vi "Voltmeter.vi"(1 "Action":T4=enum."Identify", 2 "Parameters":variant) -> (6 "Output":variant, 7 "Stop":bool)   [LabVIEW 2024]
doc: "This VI reads a single reading from a Keithley 2001 multimeter. The stop boolean is always false. If no reading is obtained a single zero is returned.\nScott Hannahs, NHMFL-FSU, Nov 1993"
uses:
  Sub Controls/Instrument Actions.ctl
  Sub Controls/Instrument Match.ctl
  Sub Controls/Public.ctl
  Sub Controls/Factory Reset.ctl
  Sub Controls/Scan Input.ctl
  Sub Controls/Scan Output.ctl
  Sub Controls/Instrument IDN.ctl
  Sub Controls/User Event Command.ctl
panel:
  in  "Factory Reset":T1
  in  "Elements":bool
  in  "Mode Sourcemeter":enum32{"Voltage", "Current", "Both"}(radio)
  out "Title":string
  in  "Public":T2
  in  "Address":u16(ring)
  out "Model":string
  in  "Instruments":T3[](array[typedef])=[{"Model"="34401", "Manufacturer"="HEWLETT-PACKARD", "Term Character"="", "Wait Time (mS)"=0, "Wait for SRQ"=FALSE, "Type"="Voltmeter"}, {"Model"="MODEL 182", "Manufacturer"="KEITHLEY INSTRUMENTS", "Term Character"="", "Wait Time (mS)"=0, "Wait for SRQ"=FALSE, "Type"="Voltmeter"}, {"Model"="MODEL 200[012]", "Manufacturer"="KEITHLEY INSTRUMENTS", "Term Character"="", "Wait Time (mS)"=0, "Wait for SRQ"=FALSE, "Type"="Voltmeter"}, {"Model"="MODEL 6221[A]*", "Manufacturer"="KEITHLEY INSTRUMENTS", "Term Character"="", "Wait Time (mS)"=0, "Wait for SRQ"=FALSE, "Type"="Voltmeter"}, {"Model"="MODEL 2420", "Manufacturer"="KEITHLEY INSTRUMENTS", "Term Character"="", "Wait Time (mS)"=0, "Wait for SRQ"=FALSE, "Type"="Voltmeter"}, {"Model"="MODEL 2182[A]*", "Manufacturer"="KEITHLEY INSTRUMENTS", "Term Character"="", "Wait Time (mS)"=0, "Wait for SRQ"=FALSE, "Type"="Voltmeter"}, {"Model"="MODEL 6517[AB]", "Manufacturer"="KEITHLEY INSTRUMENTS", "Term Character"="", "Wait Time (mS)"=0, "Wait for SRQ"=FALSE, "Type"="Electrometer"}, {"Model"="MODEL 6430", "Manufacturer"="KEITHLEY INSTRUMENTS", "Term Character"="", "Wait Time (mS)"=0, "Wait for SRQ"=FALSE, "Type"="Sourcemeter"}, {"Model"="5313[12]A", "Manufacturer"="HEWLETT-PACKARD", "Term Character"="", "Wait Time (mS)"=0, "Wait for SRQ"=FALSE, "Type"="Counter"}, {"Model"="MODEL 2450", "Manufacturer"="KEITHLEY INSTRUMENTS", "Term Character"="", "Wait Time (mS)"=0, "Wait for SRQ"=FALSE, "Type"="Sourcemeter"}, {"Model"="MODEL DMM7510", "Manufacturer"="KEITHLEY INSTRUMENTS", "Term Character"="", "Wait Time (mS)"=0, "Wait for SRQ"=FALSE, "Type"="Voltmeter"}]
  out "Measurement":dbl[](array[numeric]) format="%^_7e"
  in  "VISA resource name":refnum<visa-resource-name>
  # "Term Char"
  # "Wait Time (mS)"
  # "Wait for SRQ?"
  # "Type"
  # "Manufacturer"
  # "Model"
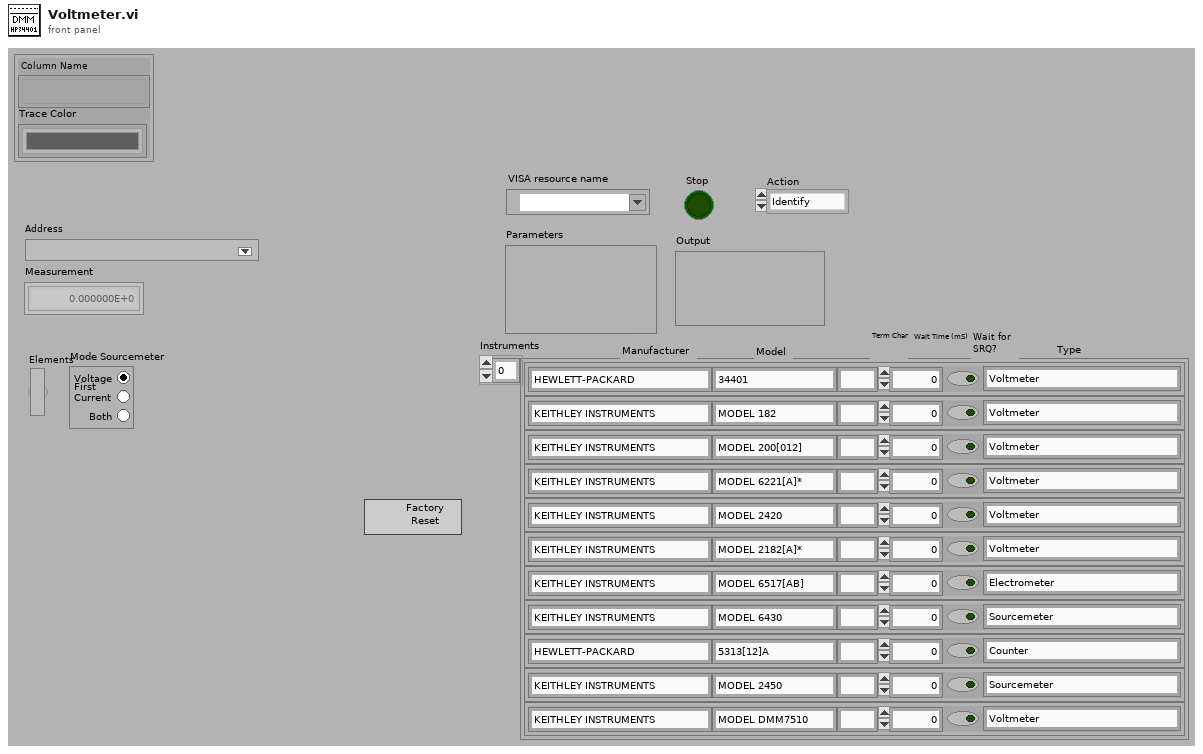
[diagram p1: front panel]
types:
  T1 = typedef "Factory Reset.ctl" = bool
  T2 = typedef "Public.ctl" = cluster{"Column Name":string[], "Trace Color":u32[]}
  T3 = typedef "Instrument Match.ctl" = cluster{"Model":string, "Manufacturer":string, "Term Character":string, "Wait Time (mS)":u32, "Wait for SRQ":bool, "Type":string}
  T4 = typedef "Instrument Actions.ctl" = enum16{"Scan", "Identify", "New", "Configure", "Initialize", "Test", "Read", "Close"}
  T5 = typedef "Scan Output.ctl" = cluster{"Manufacturer":string, "Model":string, "Info":string, "Revision":string, "error out":errorcluster}
  T6 = typedef "Scan Input.ctl" = cluster{"VISA resource name":refnum<visa-resource-name>, "ID String in":string}
  T7 = typedef "Instrument IDN.ctl" = cluster{"VISA Address":string, "Status":u16, "Manufacturer":string, "Model":string, "Info":string, "Info 2":string, "Misc Data":variant}
  T8 = typedef "User Event Command.ctl" = enum32{"Stop Config"}
  T9 = typedef "Instrument Properties.ctl" = cluster{"Public":T2, "Private":T10}
  T10 = typedef "Private.ctl" = cluster{"Path":path, "VI Refnum":T11, "Name":string, "# of Values":i32, "Scale Factors":dbl[], "Display":T12[], "Offset":dbl[]}
  T11 = typedef "Instrument Ref.ctl" = refnum<vi>
  T12 = typedef "SystemCheckBox-resize.ctl" = bool
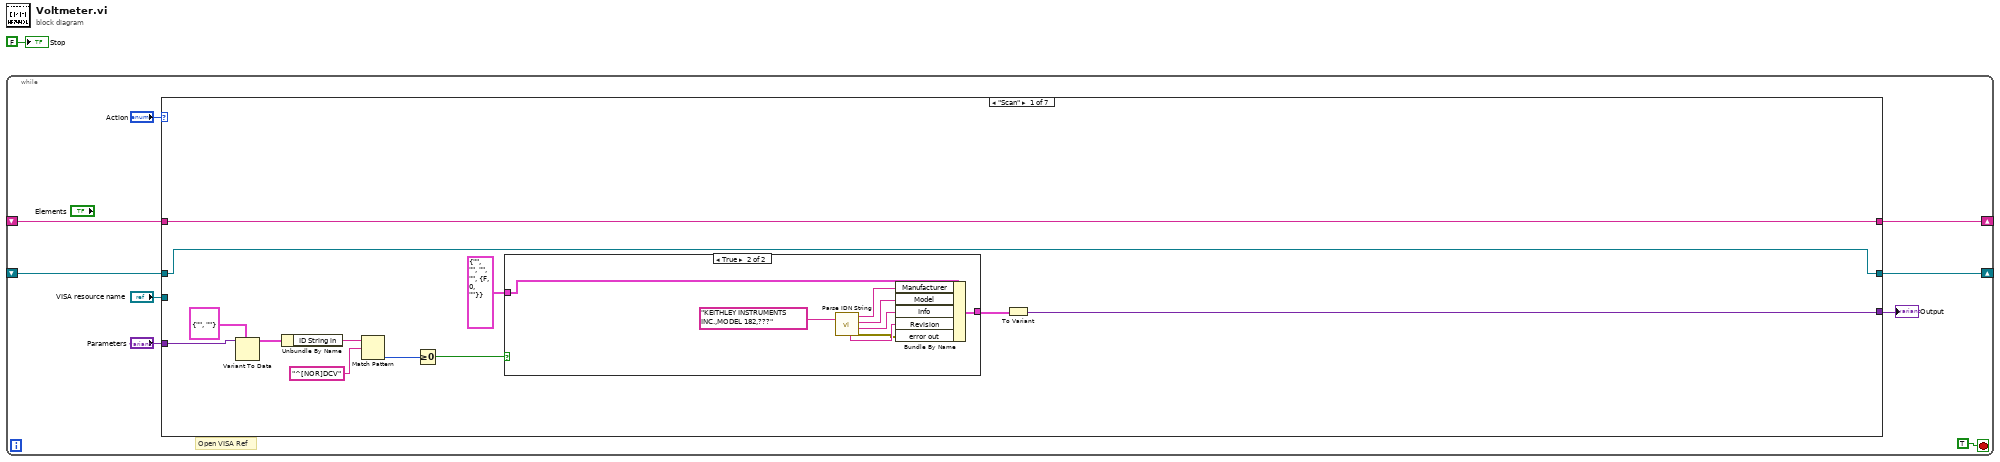
[diagram p0: block diagram]
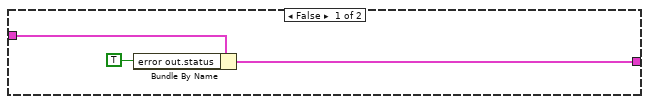
[diagram p2: hidden frame]
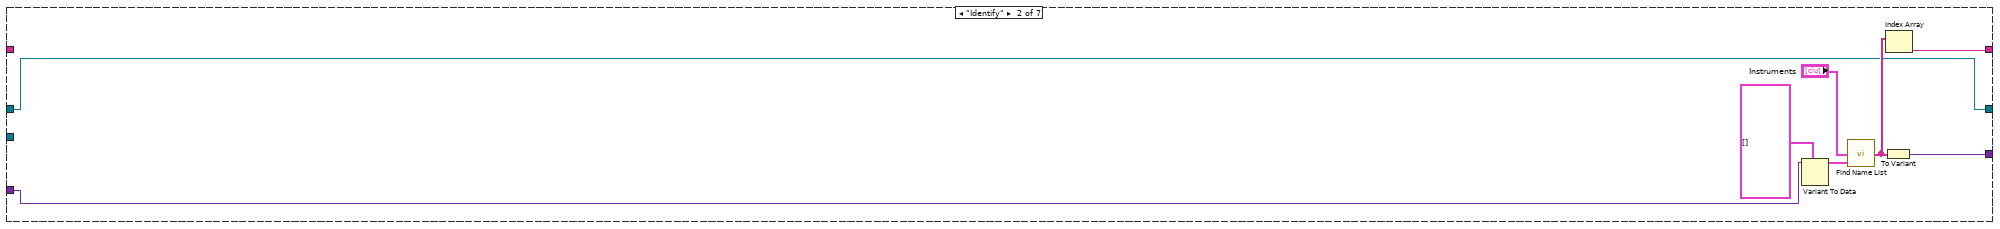
[diagram p3: hidden frame]
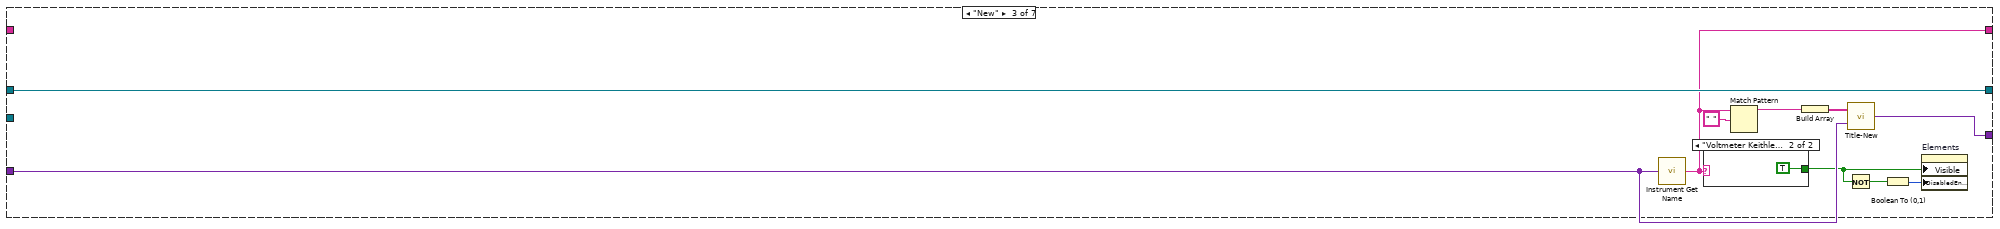
[diagram p4: hidden frame]
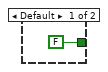
[diagram p5: hidden frame]
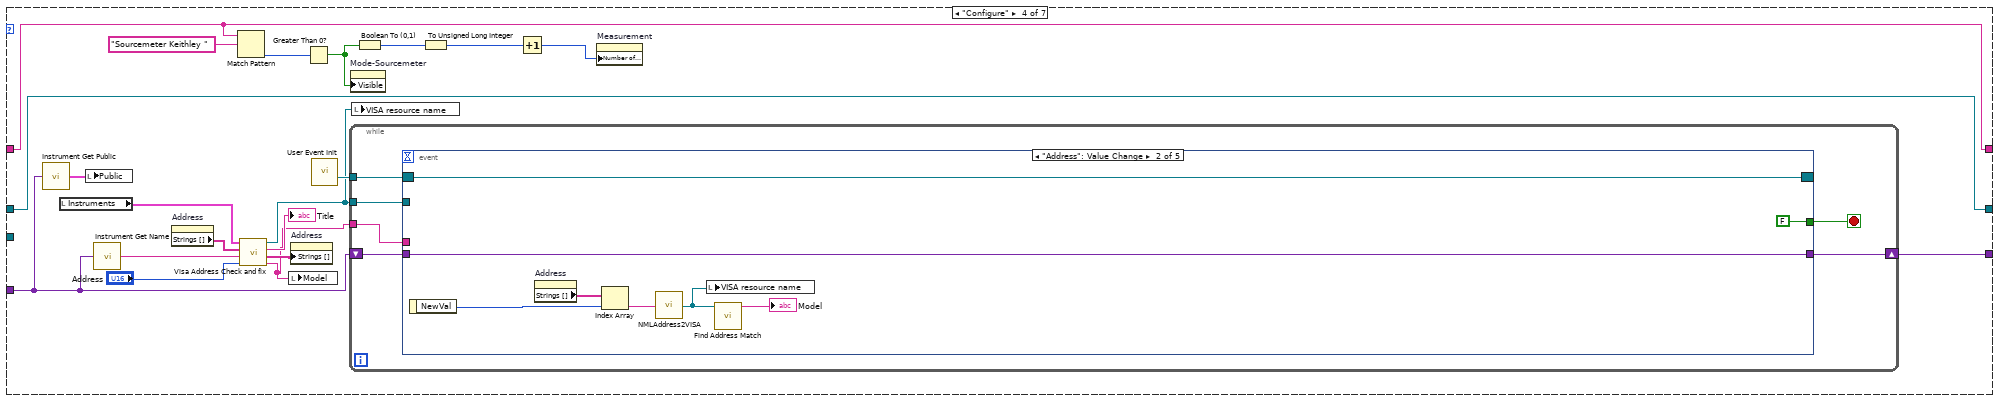
[diagram p6: hidden frame]
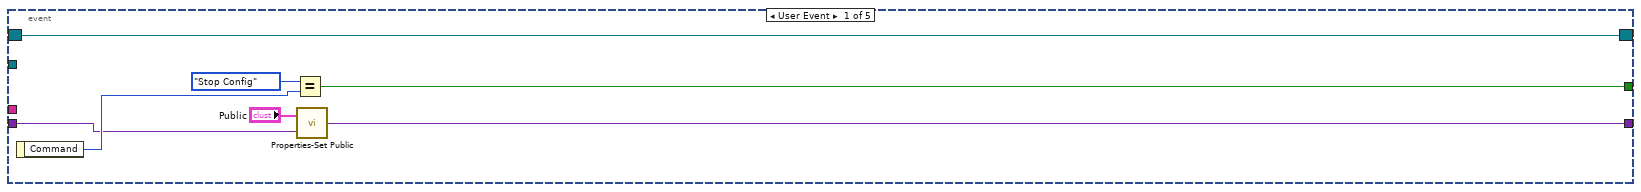
[diagram p7: hidden frame]
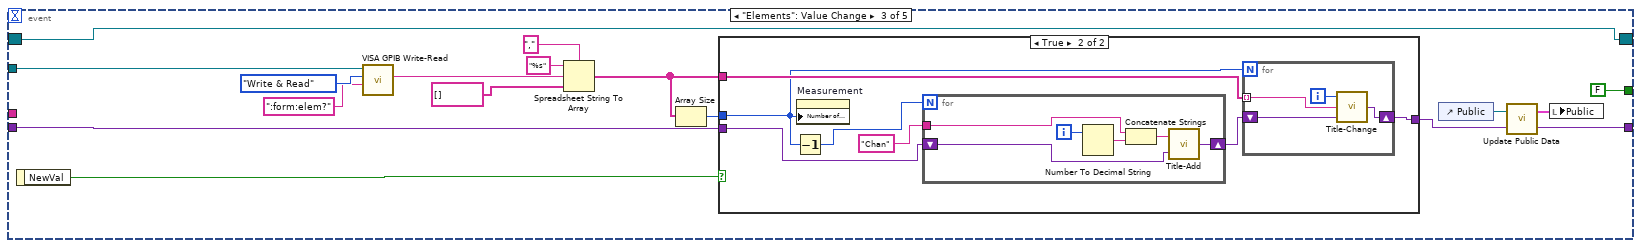
[diagram p8: hidden frame]
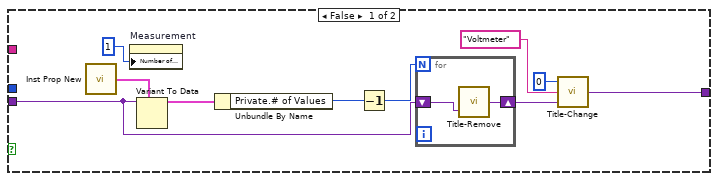
[diagram p9: hidden frame]
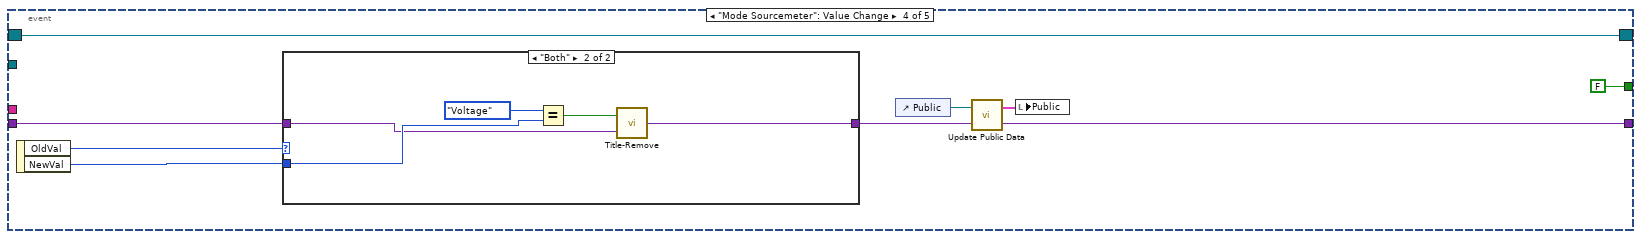
[diagram p10: hidden frame]
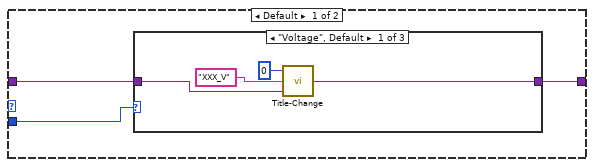
[diagram p11: hidden frame]
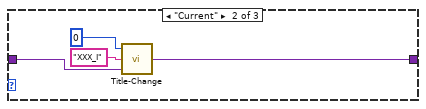
[diagram p12: hidden frame]
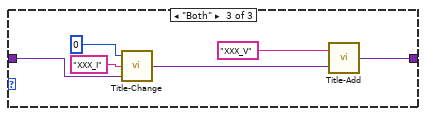
[diagram p13: hidden frame]
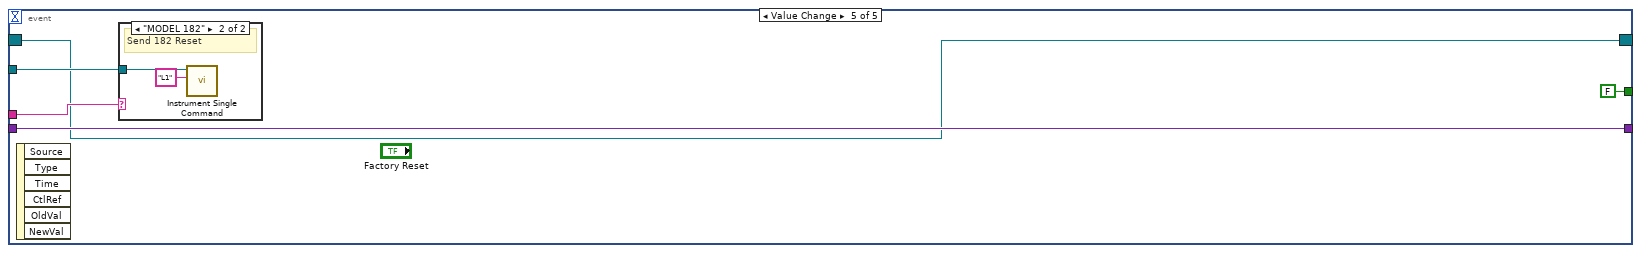
[diagram p14: hidden frame]
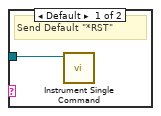
[diagram p15: hidden frame]
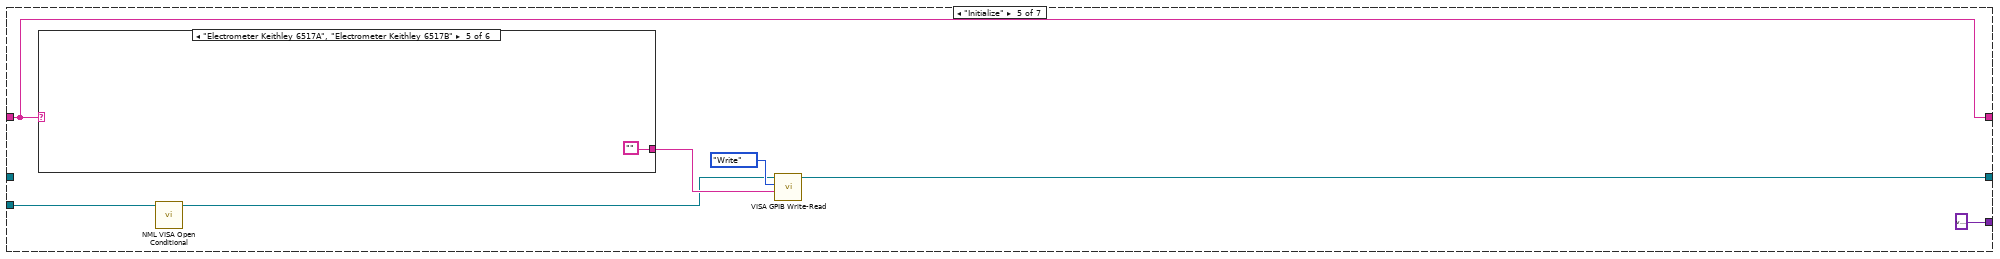
[diagram p16: hidden frame]
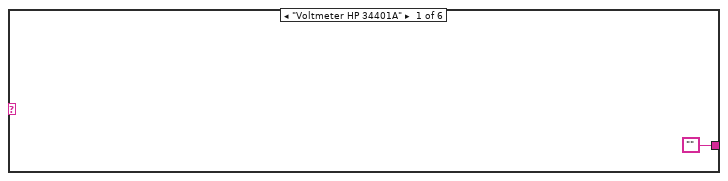
[diagram p17: hidden frame]
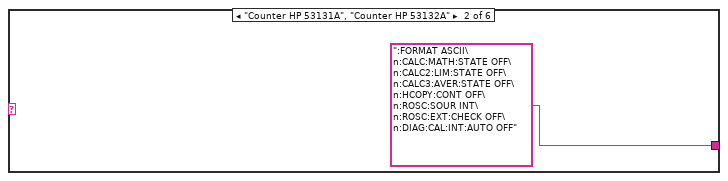
[diagram p18: hidden frame]
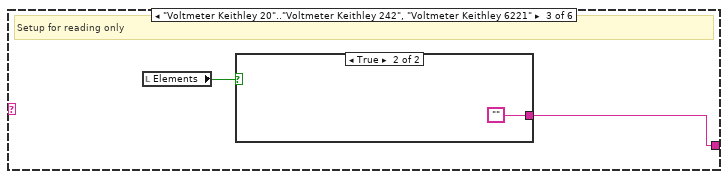
[diagram p19: hidden frame]
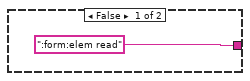
[diagram p20: hidden frame]
diagram:
  n1 = while {
    shift-right: [w6] -> _
    shift-left: _ -> [w5]
    shift-right: [w3] -> _
    shift-left: _ -> [w2]
    stop <- TRUE stop-if-true
    # "Open VISA Ref"
    n2 = case shown="\"Scan\"" "Action" {
      tunnel: [w15 w41 w51 w68 variant ("Variant") w203 variant ("Variant")] -> w8
      tunnel: "VISA resource name" -> [_ _ _ _ w186 _ _]
      tunnel: [w14 w36 w45 w59 w183 w197 w240] -> w6
      tunnel: w5 -> [w14 _ _ w59 w183 w197 w240]
      tunnel: "Parameters" -> [w22 w40 w49 w65 _ _ _]
      tunnel: [w11 w34 w50 w66 w182 w201 refnum<visa-resource-name> refnum ("Open VISA Resource name")] -> w3
      tunnel: w2 -> [w11 w34 w50 w66 _ w202 w238]
      frame "Scan" {
        n3 = Variant To Data(type=T6 {"VISA resource name"="", "ID String in"=""} ("Scan Input"), Variant=w22) -> (data=w20:T6)  [unwired: 1 in, 1 out]
        n4 = Unbundle By Name(w20) -> ("ID String in"=w17:string)
        n5 = Match Pattern(string=w17, regular expression="^[NOR]DCV") -> (offset past match=w19:i32)  [unwired: 1 in, 3 out]
        n6 = Greater Or Equal To 0?(x=w19) -> (x >= 0?=w16:bool)
        n7 = case shown="True" w16 {
          tunnel: T5 {"Manufacturer"="", "Model"="", "Info"="", "Revision"="", "error out"={"status"=FALSE, "code"=0, "source"=""}} ("Scan Output") -> [w24 w33]
          tunnel: [w25 w32] -> w12
          frame False {
            n8 = Bundle By Name(cluster=w24, "error out.status"=TRUE) -> (w25:T5)
          }
          frame True {
            n9 = call "Parse IDN String.vi"("IDN String"="KEITHLEY INSTRUMENTS INC.,MODEL 182,???") -> ("error out"=w29:errorcluster, "Info"=w28:string, "Model"=w27:string, "Manufacturer"=w26:string, "Revision"=w30:string)  [unwired: 1 in]
            n10 = Bundle By Name(cluster=w33, "Manufacturer"=w26, "Model"=w27, "Info"=w28, "Revision"=w30, "error out"=w29) -> (w32:T5)
          }
        }
        n11 = To Variant(anything=w12) -> (Variant=w15:variant)
      }
      frame "Identify" {
        n12 = Variant To Data(type=T7[] [], Variant=w40) -> (data=w38:T7[])  [unwired: 1 in, 1 out]
        n13 = call "Find Name List.vi"("Bus Scan"=w38, "Instruments"="Instruments") -> ("Names"=w35:string[])  [unwired: 1 in]
        n14 = Index Array(array=w35) -> (element=w36:string)  [unwired: 1 in]
        n15 = To Variant(anything=w35) -> (Variant=w41:variant)
      }
      frame "New" {
        n16 = call "Instrument Get Name.vi"("Parameters"=w49) -> ("Type"=w45:string)
        n17 = case shown="\"Voltmeter Keithley 6221\"" w45 {
          tunnel: [FALSE ("Visible") TRUE ("Visible")] -> w44
          frame Default {
          }
          frame "Voltmeter Keithley 6221" {
          }
        }
        n18 = Match Pattern(string=w45, regular expression=" ") -> (before substring=w47:string)  [unwired: 1 in, 3 out]
        n19 = Build Array(w47) -> (w48:string[])
        n20 = Not(x=w44) -> (.not. x?=w42:bool)
        n21 = call "Title-New.vi"("Parameters"=w49, "Array"=w48) -> ("Instrument Prop"=w51:variant)
        n22 = Boolean To (0,1)(Boolean=w42) -> (0, 1=w43:i16)
        n23 = property on="Elements" class="Bool (strict)"("Visible"=w44, "DisabledEnum"=w43) -> ()  [unwired: 2 in, 2 out]
      }
      frame "Configure" {
        n24 = call "Instrument Get Public.vi"("Variant"=w65) -> ("Public"=w69:T2)
        n25 = local read "Instruments"() -> (w70:T3[])
        n26 = local write "Public"(w69) -> ()
        n27 = call "Instrument Get Name.vi"("Parameters"=w65) -> ("Type"=w64:string)
        n28 = property on="Address" class="Ring (strict)"() -> ("Strings []"=w71:string[])  [unwired: 2 in, 2 out]
        n29 = Match Pattern(string=w59, regular expression="Sourcemeter Keithley " ("y")) -> (offset past match=w57:i32)  [unwired: 1 in, 3 out]
        n30 = call "Visa Address Check and fix.vi"("Address"="Address", "Name"=w64, "NML Addresses"=w71, "Instruments"=w70) -> ("Model"=w54:string, "NML Addresses"=w73:string[], "Title"=→"Title":string, "VISA resource name"=w55:refnum<visa-resource-name>)  [unwired: 2 out]
        n31 = local write "Model"(w54) -> ()
        n32 = property on="Address" class="Ring (strict)"("Strings []"=w73) -> ()  [unwired: 2 in, 2 out]
        n33 = Greater Than 0?(x=w57) -> (x > 0?=w56:bool)
        n34 = call "User Event Init.vi"() -> ("Event Registration Refnum"=w67:refnum<event-registration>)  [unwired: 14 in, 1 out]
        n35 = while {
          tunnel: w67 -> [w76]
          shift-right: [w79] -> w68
          shift-left: w65 -> [w77]
          tunnel: w55 -> [w75]
          tunnel: w54 -> [w74]
          stop <- w78 stop-if-true
          n36 = event shown="[1] \"Address\": Value Change" {
            selector: w76 -> [w80 w88 w108 w149 w172]
            dyn-events: [w80 w88 w108 w149 w172] -> _
            timeout: _ -> [_ _ _ _ _]
            tunnel: [w84 w89 w105 w143 w174] -> w79
            tunnel: [w82 FALSE FALSE FALSE FALSE] -> w78
            tunnel: w77 -> [w85 w89 w111 w145 w174]
            tunnel: w75 -> [_ _ w101 _ w176]
            tunnel: w74 -> [_ _ _ _ w175]
            event User Event {
              n37 = event-data() -> ("Command"=w86:T8)  [unwired: 1 in]
              n38 = Equal?(x=User_Event_Command."Stop Config", y=w86) -> (x = y?=w82:bool)
              n39 = call "Properties-Set Public.vi"("Variant"=w85, "New Public"="Public") -> ("Variant 2"=w84:variant)
            }
            event "Address": Value Change {
              n40 = event-data() -> ("NewVal"=w94:u16)  [unwired: 1 in]
              n41 = property on="Address" class="Ring (strict)"() -> ("Strings []"=w91:string[])  [unwired: 2 in, 2 out]
              n42 = Index Array(array=w91, index=w94) -> (element=w92:string)
              n43 = call "NMLAddress2VISA.vi"("NML Address"=w92) -> ("VISA resource name"=w87:refnum<visa-resource-name>)
              n44 = local write "VISA resource name"(w87) -> ()
              n45 = call "Find Address Match.vi"("VISA resource name"=w87) -> ("Model"=→"Model":string)  [unwired: 3 in, 3 out]
            }
            event "Elements": Value Change {
              n46 = event-data() -> ("NewVal"=w110:bool)  [unwired: 1 in]
              n47 = call "VISA GPIB Write-Read.vi"("Command"=":form:elem?", "Action"=enum16{"Write", "Read", "Write & Read"}."Write & Read", "VISA resource name"=w101) -> ("String Returned"=w100:string)  [unwired: 5 in, 3 out]
              n48 = Spreadsheet String To Array(delimiter (Tab)=",", format string="%s", spreadsheet string=w100, array type (2D Dbl)=string[] [] ("array")) -> (array=w95:string[])
              n49 = Array Size(array=w95) -> (size(s)=w97:i32)
              n50 = case shown="True" w110 {
                tunnel: w111 -> [w118 w129]
                tunnel: [w115 w125] -> w106
                tunnel: w97 -> [_ w126]
                tunnel: w95 -> [_ w127]
                frame False {
                  n51 = call "Inst Prop New.vi"() -> ("Instrument Prop Out"=w121:T9)
                  n52 = property on="Measurement" class="Arr (strict)"("Number of Columns"=u32 1) -> ()  [unwired: 2 in, 2 out]
                  n53 = Variant To Data(type=w121, Variant=w118) -> (data=w120:T9)  [unwired: 1 in, 1 out]
                  n54 = Unbundle By Name(w120) -> ("Private.# of Values"=w119:i32)
                  n55 = Decrement(x=w119) -> (x-1=w113:i32)
                  n56 = for {
                    N: w113 -> [_]
                    shift-right: [w123] -> w116
                    shift-left: w118 -> [w122]
                    n57 = call "Title-Remove.vi"("Parameters"=w122) -> ("Variant"=w123:variant)  [unwired: 1 in]
                  }
                  n58 = call "Title-Change.vi"("Parameters"=w116, "New Title"="Voltmeter", "Index"=0) -> ("Variant"=w115:variant)
                }
                frame True {
                  n59 = Decrement(x=w126) -> (x-1=w130:i32)
                  n60 = property on="Measurement" class="Arr (strict)"("Number of Columns"=w126) -> ()  [unwired: 2 in, 2 out]
                  n61 = for {
                    N: w130 -> [_]
                    tunnel: "Chan" ("String") -> [w139]
                    shift-right: [w140] -> w124
                    shift-left: w129 -> [w135]
                    i -> [w137]
                    n62 = Number To Decimal String(number=w137) -> (decimal integer string=w136:string)  [unwired: 1 in]
                    n63 = Concatenate Strings(w139, w136) -> (w138:string)
                    n64 = call "Title-Add.vi"("Parameters"=w135, "String"=w138) -> ("Variant"=w140:variant)
                  }
                  n65 = for {
                    N: w126 -> [_]
                    tunnel: w127 -> [w133] mode=indexing
                    shift-right: [w132] -> w125
                    shift-left: w124 -> [w131]
                    i -> [w134]
                    n66 = call "Title-Change.vi"("Parameters"=w131, "New Title"=w133, "Index"=w134) -> ("Variant"=w132:variant)
                  }
                }
              }
              n67 = control-ref of="Public"() -> (w104:refnum<vi>)
              n68 = call "Update Public Data.vi"("Variant In"=w106, "Public 2"=w104) -> ("Variant Out"=w105:variant, "Public"=w107:T2)
              n69 = local write "Public"(w107) -> ()
            }
            event "Mode Sourcemeter": Value Change {
              n70 = event-data() -> ("OldVal"=w147:enum32{"Voltage", "Current", "Both"}, "NewVal"=w146:enum32{"Voltage", "Current", "Both"})  [unwired: 1 in]
              n71 = case shown="\"Both\"" w147 {
                tunnel: w146 -> [w152 w170]
                tunnel: w145 -> [w151 w167]
                tunnel: [w150 w171] -> w144
                frame Default {
                  n72 = case shown="\"Voltage\", Default" w152 {
                    tunnel: w151 -> [w156 w157 w164]
                    tunnel: [w153 w158 w162] -> w150
                    frame "Voltage", Default {
                      n73 = call "Title-Change.vi"("Parameters"=w156, "New Title"="XXX_V", "Index"=0) -> ("Variant"=w153:variant)
                    }
                    frame "Current" {
                      n74 = call "Title-Change.vi"("Parameters"=w157, "New Title"="XXX_I", "Index"=0) -> ("Variant"=w158:variant)
                    }
                    frame "Both" {
                      n75 = call "Title-Change.vi"("Parameters"=w164, "New Title"="XXX_I", "Index"=0) -> ("Variant"=w163:variant)
                      n76 = call "Title-Add.vi"("Parameters"=w163, "String"="XXX_V") -> ("Variant"=w162:variant)
                    }
                  }
                }
                frame "Both" {
                  n77 = Equal?(x=enum32{"Voltage", "Current", "Both"}."Voltage", y=w170) -> (x = y?=w168:bool)
                  n78 = call "Title-Remove.vi"("Parameters"=w167, "Remove First"=w168) -> ("Variant"=w171:variant)
                }
              }
              n79 = control-ref of="Public"() -> (w141:refnum<vi>)
              n80 = call "Update Public Data.vi"("Variant In"=w144, "Public 2"=w141) -> ("Variant Out"=w143:variant, "Public"=w142:T2)
              n81 = local write "Public"(w142) -> ()
            }
            event Value Change {
              n82 = event-data() -> ()  [unwired: 1 in, 6 out]
              n83 = case shown="\"MODEL 182\"" w175 {
                tunnel: w176 -> [w177 w179]
                frame Default {
                  # "Send Default \"*RST\""
                  n84 = call "Instrument Single Command.vi"("VISA Name"=w177) -> ()  [unwired: 10 in, 1 out]
                }
                frame "MODEL 182" {
                  # "Send 182 Reset"
                  n85 = call "Instrument Single Command.vi"("Reset Command"="L1", "VISA Name"=w179) -> ()  [unwired: 9 in, 1 out]
                }
              }
            }
          }
        }
        n86 = property on="Mode-Sourcemeter" class="RadioBtnsControl (strict)"("Visible"=w56) -> ()  [unwired: 2 in, 2 out]
        n87 = local write "VISA resource name"(w55) -> ()
        n88 = Boolean To (0,1)(Boolean=w56) -> (0, 1=w62:i16)
        n89 = To Unsigned Long Integer(number=w62) -> (unsigned 32bit integer=w60:u32)
        n90 = Increment(x=w60) -> (x+1=w61:u32)
        n91 = property on="Measurement" class="Arr (strict)"("Number of Columns"=w61) -> ()  [unwired: 2 in, 2 out]
      }
      frame "Initialize" {
        n92 = case shown="\"Electrometer Keithley 6517A\", \"Electrometer Keithley 6517B\"" w183 {
          tunnel: ["" ":FORMAT ASCII\n:CALC:MATH:STATE OFF\n:CALC2:LIM:STATE OFF\n:CALC3:AVER:STATE OFF\n:HCOPY:CONT OFF\n:ROSC:SOUR INT\n:ROSC:EXT:CHECK OFF\n:DIAG:CAL:INT:AUTO OFF" w190 ":form:elem VOLT,CURR" "" ""] -> w184
          frame "Voltmeter HP 34401A" {
          }
          frame "Counter HP 53131A", "Counter HP 53132A" {
          }
          frame "Voltmeter Keithley 20".."Voltmeter Keithley 242", "Voltmeter Keithley 6221" {
            # "Setup for reading only"
            n93 = local read "Elements"() -> (w189:bool)
            n94 = case shown="True" w189 {
              tunnel: [":form:elem read" ""] -> w190
              frame False {
              }
              frame True {
              }
            }
          }
          frame "Sourcemeter Keithley 6430" {
          }
          frame "Electrometer Keithley 6517A", "Electrometer Keithley 6517B" {
          }
          frame "Voltmeter Keithley 182", Default {
          }
        }
        n95 = call "NML VISA Open Conditional.vi"("VISA resource name"=w186) -> ("dup VISA Session"=w180:refnum<visa-resource-name>)  [unwired: 8 in, 2 out]
        n96 = call "VISA GPIB Write-Read.vi"("Command"=w184, "Action"=enum16{"Write", "Read", "Write & Read"}."Write", "VISA resource name"=w180) -> ("dup VISA Session"=w182:refnum<visa-resource-name>)  [unwired: 5 in, 3 out]
      }
      frame "Test", "Read" {
        n97 = case shown="\"Sourcemeter Keithley 2450\"" w197 {
          tunnel: ["read?" "fetc?" "Sens:data:latest?" w219 w229 ""] -> w200
          tunnel: [u32 0 ("wait (mS)") u32 50 ("wait (mS)") u32 0 ("wait (mS)") u32 0 ("wait (mS)") u32 0 ("wait (mS)") u32 0 ("wait (mS)")] -> w196
          frame "Voltmeter HP 34401A", "Voltmeter Keithley DMM7510" {
          }
          frame "Counter HP 53131A", "Counter HP 53132A" {
          }
          frame "Electrometer Keithley 6517A", "Electrometer Keithley 6517B", "Voltmeter Keithley 2".."Voltmeter Keithley 25", "Voltmeter Keithley 6221" {
          }
          frame "Sourcemeter Keithley 6430" {
            n98 = Not Equal?(x="Mode Sourcemeter", y=enum32{"Voltage", "Current", "Both"}."Current") -> (x != y?=w223:bool)
            n99 = Select(t=":meas:volt?", s=w223, f="") -> (s? t:f=w221:string)
            n100 = Concatenate Strings(":meas:curr?;", w221) -> (w219:string)
          }
          frame "Sourcemeter Keithley 2450" {
            n101 = local read "Mode Sourcemeter"() -> (w227:enum32{"Voltage", "Current", "Both"})
            n102 = Not Equal?(x=w227, y=enum32{"Voltage", "Current", "Both"}."Current") -> (x != y?=w233:bool)
            n103 = Select(t=":meas:volt?;", s=w233, f="") -> (s? t:f=w231:string)
            n104 = Concatenate Strings(w231, ":meas:curr?") -> (w229:string)
          }
          frame "Voltmeter Keithley 182", Default {
          }
        }
        n105 = call "General VISA transaction.vi"("Wait (mS)"=w196, "Command String"=w200, "VISA Session"=w202) -> ("Measurement"=w199:dbl[], "dup VISA Session"=w201:refnum<visa-resource-name>)  [unwired: 3 in, 4 out]
        n106 = case shown="\"Sourcemeter Keithley 2450\"" w197 {
          tunnel: [w204 w208 w211] -> w198
          tunnel: w199 -> [w204 w209 w210]
          frame Default {
          }
          frame "Sourcemeter Keithley 6430" {
            n107 = Index Array(array=w209, index #1=0 ("index")) -> (element #2=w207:dbl, element #3=w206:dbl)  [unwired: 3 in, 2 out]
            n108 = Build Array(w207, w206) -> (w208:dbl[])
          }
          frame "Sourcemeter Keithley 2450" {
            n109 = Reverse 1D Array(array=w210) -> (reversed array=w211:dbl[])
          }
        }
        "Measurement" <- w198
        n110 = To Variant(anything=w198) -> (Variant=w203:variant)
      }
      frame "Close" {
        n111 = call "NML VISA Close.vi"("VISA resource name"=w238) -> ()  [unwired: 10 in, 1 out]
      }
    }
    "Output" <- w8
  }
  "Stop" <- FALSE ("Stop")
